vi "Fgen Module.vi"() -> ()   [LabVIEW 2021]
uses:
  <instrlib>/niDMM/nidmm.llb/niDMM Configure Measurement Digits.vi
  <instrlib>/niDMM/nidmm.llb/niDMM Resolution in Digits.ctl
  <instrlib>/niDMM/nidmm.llb/niDMM Function.ctl
panel:
  out "Measurement":dbl format="%.6p"
  in  "Range":dbl=10.0 format="%.2f"
  in  "Device Name":refnum<k15>="Dev1"
  out "Signal Out of Range":bool
  in  "Measurement Type":T1
  out "Absolute Resolution":dbl format="%#_3p"
  in  "Resolution in Digits":T2=5.5 items=["3 1/2"=3.5, "4 1/2"=4.5, "5 1/2"=5.5, "6 1/2"=6.5, "7 1/2"=7.5]
  in  "duration":dbl
  out "Actual Duration":dbl
  in  "I2C Generator Fgen":refnum<k15>
  in  "amplitude":dbl=6.0
  in  "frequency":dbl=6.0
  in  "waveform":T3(ring)=enum."Noise"
  in  "I2C Generator Fgen Channel":string
  out "error out":errorcluster
  in  "error in":errorcluster
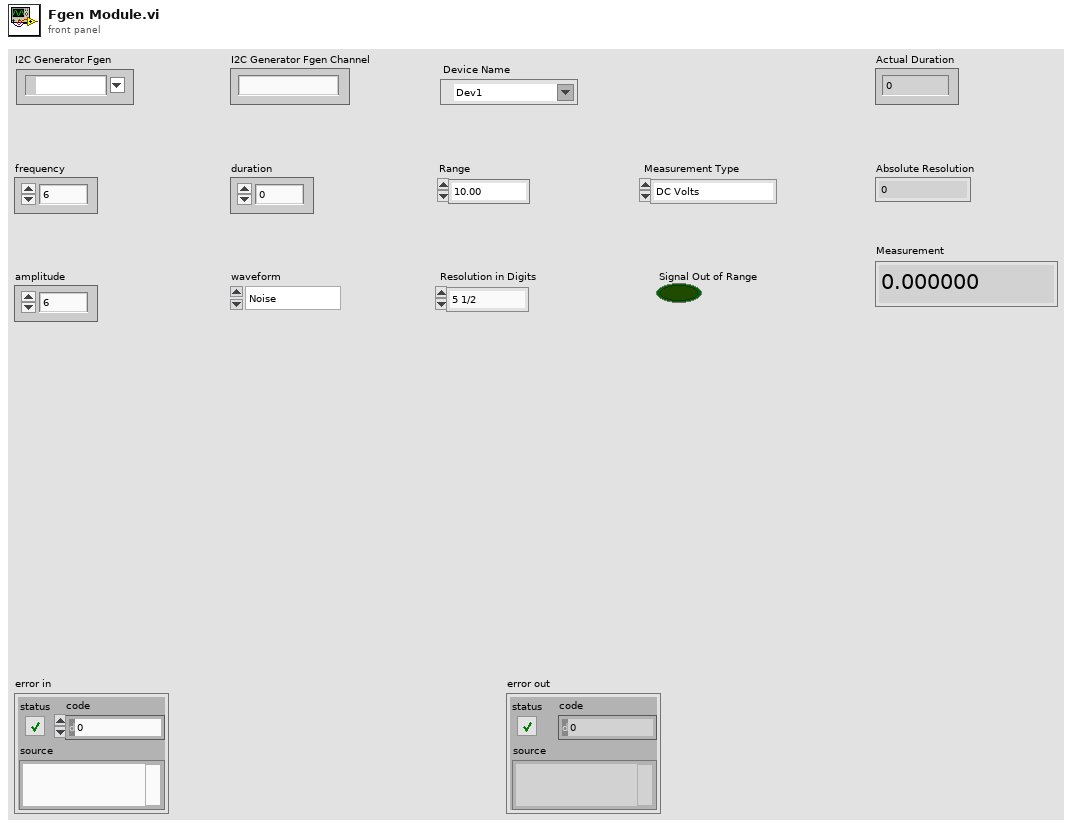
[diagram p1: front panel]
types:
  T1 = typedef "niDMM Function.ctl" = enum16{"DC Volts", "AC Volts", "DC Current", "AC Current", "2-wire Resistance", "4-wire Resistance", "Diode", "Frequency", "Period", "AC Volts DC Coupled", "Capacitance", "Inductance", "Temperature"}
  T2 = typedef "niDMM Resolution in Digits.ctl" = dbl
  T3 = enum32{"Sine", "Square", "Triangle", "Ramp Up", "Ramp Down", "DC", "Noise", "User"}
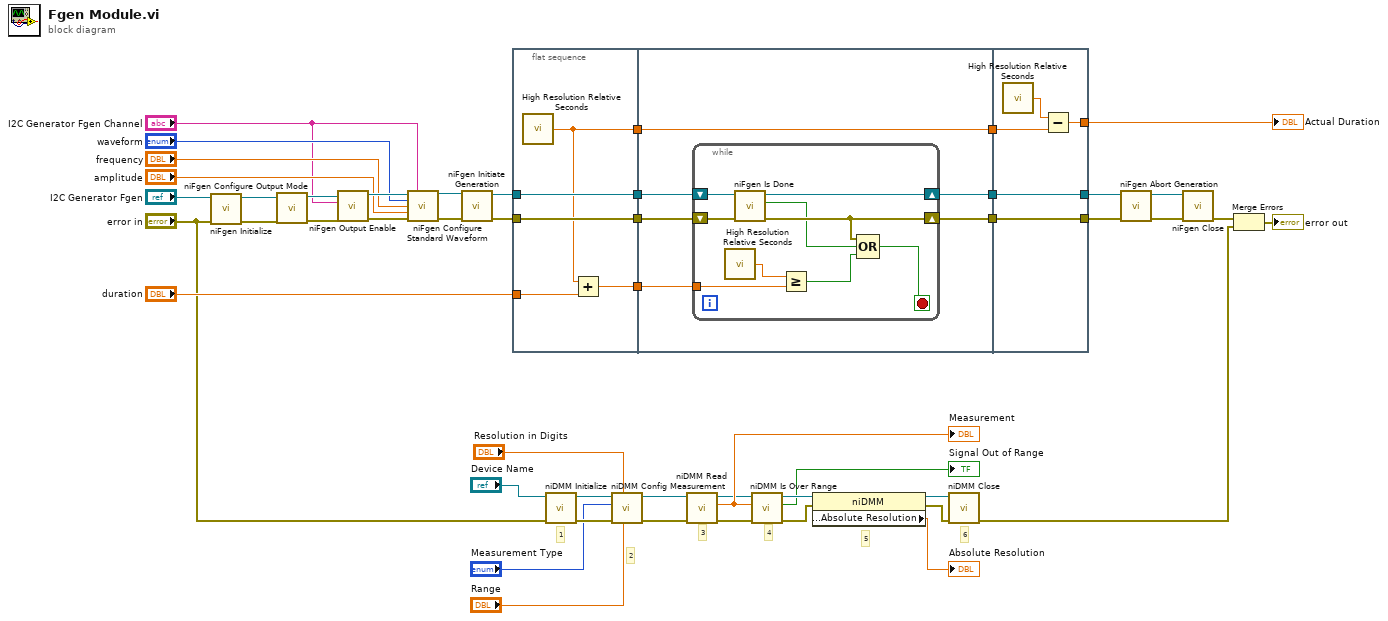
[diagram p0: block diagram]
diagram:
  # "2"
  # "1"
  # "6"
  # "5"
  # "4"
  # "3"
  n1 = call <instrlib>:"niFgen Initialize.vi"("error in (no error)"="error in", "Resource Name"="I2C Generator Fgen") -> ("error out"=w46:errorcluster, "Instrument Handle Out"=w49:refnum<k15>)  [unwired: 8 in]
  n2 = call <instrlib>:"niFgen Configure Output Mode.vi"("error in (no error)"=w46, "Instrument Handle"=w49) -> ("error out"=w35:errorcluster, "Instrument Handle Out"=w45:refnum<k15>)  [unwired: 7 in]
  n3 = call <instrlib>:"niFgen Output Enable.vi"("error in (no error)"=w35, "Channel Name"="I2C Generator Fgen Channel", "Instrument Handle"=w45) -> ("error out"=w47:errorcluster, "Instrument Handle Out"=w44:refnum<k15>)  [unwired: 7 in]
  n4 = call <instrlib>:"niFgen Configure Standard Waveform.vi"("Instrument Handle"=w44, "Channel Name"="I2C Generator Fgen Channel", "Waveform"="waveform", "Frequency"="frequency", "Amplitude"="amplitude", "error in (no error)"=w47) -> ("Instrument Handle Out"=w43:refnum<k15>, "error out"=w48:errorcluster)  [unwired: 8 in]
  n5 = call <instrlib>:"niFgen Initiate Generation.vi"("error in (no error)"=w48, "Instrument Handle"=w43) -> ("error out"=w40:errorcluster, "Instrument Handle Out"=w42:refnum<k15>)  [unwired: 8 in]
  n6 = flat-sequence {
    tunnel: w40 -> [w53]
    tunnel: w42 -> [w54]
    tunnel: [w54] -> w29
    tunnel: [w53] -> w28
    tunnel: [w52] -> w24
    tunnel: "duration" -> [w51]
    tunnel: [w50] -> w21
    tunnel: w29 -> [w60]
    tunnel: w28 -> [w58]
    tunnel: [w59] -> w27
    tunnel: [w57] -> w26
    tunnel: [w56] -> w25
    tunnel: w24 -> [w56]
    tunnel: w21 -> [w55]
    tunnel: [w73] -> w39
    tunnel: [w74] -> w41
    tunnel: w27 -> [w74]
    tunnel: w26 -> [w73]
    tunnel: w25 -> [w71]
    tunnel: [w70] -> w23
    frame #0 {
      n7 = call <vilib>:"High Resolution Relative Seconds.vi"() -> ("relative seconds"=w52:dbl)
      n8 = Add(x=w52, y=w51) -> (x+y=w50:dbl)
    }
    frame #1 {
      n9 = while {
        shift-right: [w68] -> w59
        shift-left: w60 -> [w69]
        shift-right: [w66] -> w57
        shift-left: w58 -> [w67]
        tunnel: w55 -> [w63]
        stop <- w65 stop-if-true
        n10 = call <vilib>:"High Resolution Relative Seconds.vi"() -> ("relative seconds"=w64:dbl)
        n11 = call <instrlib>:"niFgen Is Done.vi"("error in (no error)"=w67, "Instrument Handle"=w69) -> ("error out"=w66:errorcluster, "Done"=w61:bool, "Instrument Handle Out"=w68:refnum<k15>)  [unwired: 7 in]
        n12 = Greater Or Equal?(x=w64, y=w63) -> (x >= y?=w62:bool)
        n13 = Compound Arithmetic op=OR(w66, w61, w62) -> (w65:bool)
      }
    }
    frame #2 {
      n14 = call <vilib>:"High Resolution Relative Seconds.vi"() -> ("relative seconds"=w72:dbl)
      n15 = Subtract(x=w72, y=w71) -> (x-y=w70:dbl)
    }
  }
  n16 = call <instrlib>:"niDMM Initialize.vi"("error in (no error)"="error in", "Instrument Descriptor"="Device Name") -> ("error out"=w13:errorcluster, "instrument handle out"=w14:refnum<k15>)  [unwired: 8 in]
  n17 = call-poly <instrlib>:"niDMM Config Measurement.vi"("Range"="Range", "Resolution in Digits"="Resolution in Digits", "error in (no error)"=w13, "Function"="Measurement Type", "instrument handle"=w14) -> ("error out"=w6:errorcluster, "instrument handle out"=w7:refnum<k15>)  [unwired: 5 in]
  n18 = call <instrlib>:"niDMM Read.vi"("error in (no error)"=w6, "instrument handle"=w7) -> ("error out"=w9:errorcluster, "Measurement"=w11:dbl, "instrument handle out"=w8:refnum<k15>)  [unwired: 7 in]
  "Measurement" <- w11
  n19 = call <instrlib>:"niDMM Is Over Range.vi"("error in (no error)"=w9, "Measurement"=w11, "instrument handle"=w8) -> ("error out"=w17:errorcluster, "Over Range?"=→"Signal Out of Range":bool, "instrument handle out"=w15:refnum<k15>)  [unwired: 6 in]
  n20 = property class="niDMM"(reference=w15, error in=w17) -> (reference out=w16:refnum<k15>, error out=w18:errorcluster, "Configuration:Absolute Resolution"=→"Absolute Resolution":dbl)
  n21 = call <instrlib>:"niDMM Close.vi"("error in (no error)"=w18, "instrument handle"=w16) -> ("error out"=w2:errorcluster)  [unwired: 9 in]
  n22 = call <instrlib>:"niFgen Abort Generation.vi"("error in (no error)"=w39, "Instrument Handle"=w41) -> ("error out"=w37:errorcluster, "Instrument Handle Out"=w38:refnum<k15>)  [unwired: 8 in]
  n23 = call <instrlib>:"niFgen Close.vi"("error in (no error)"=w37, "Instrument Handle"=w38) -> ("error out"=w36:errorcluster)  [unwired: 9 in]
  n24 = Merge Errors(w36, w2) -> (→"error out":errorcluster)
  "Actual Duration" <- w23
